vi "Are We Calibrating Steering.vi"() -> ()   [LabVIEW 2012]
panel:
  out "Are We Calibrating Steering?":bool
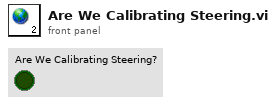
[diagram p1: front panel]
diagram:
